vi "sub_LF_params.vi"(6 "error in (no error)":errorcluster, 8 "Numeric":u32, 9 "LightField Automation in":refnum<class "LightField Automation.lvclass">) -> (0 "error out":errorcluster, 2 "Params CCD":string, 3 "LightField Automation out":refnum<class "LightField Automation.lvclass">)   [LabVIEW 2019]
doc: "Runs the Winx32 software trough Labview.\nSoftware trigger with Notifu Winx_Start\nAbort with Notify Winx_Abort\nMade by Wim van Dieren, ImSpec"
uses:
  Ligth Field/lightfield-automation-labview/LightField Automation.lvclass
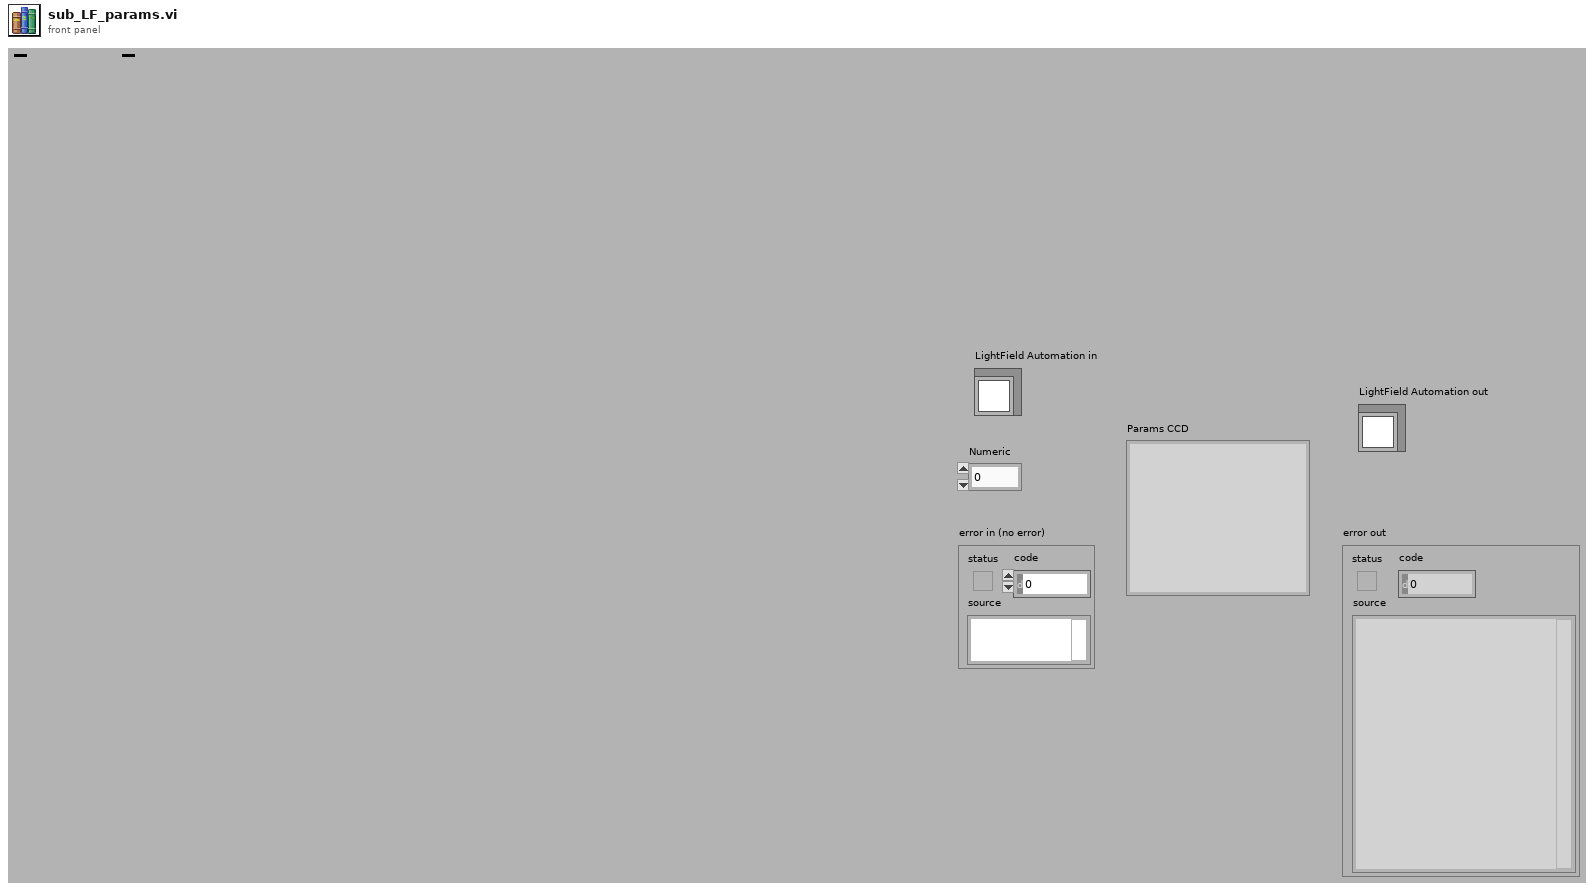
[diagram p1: front panel]
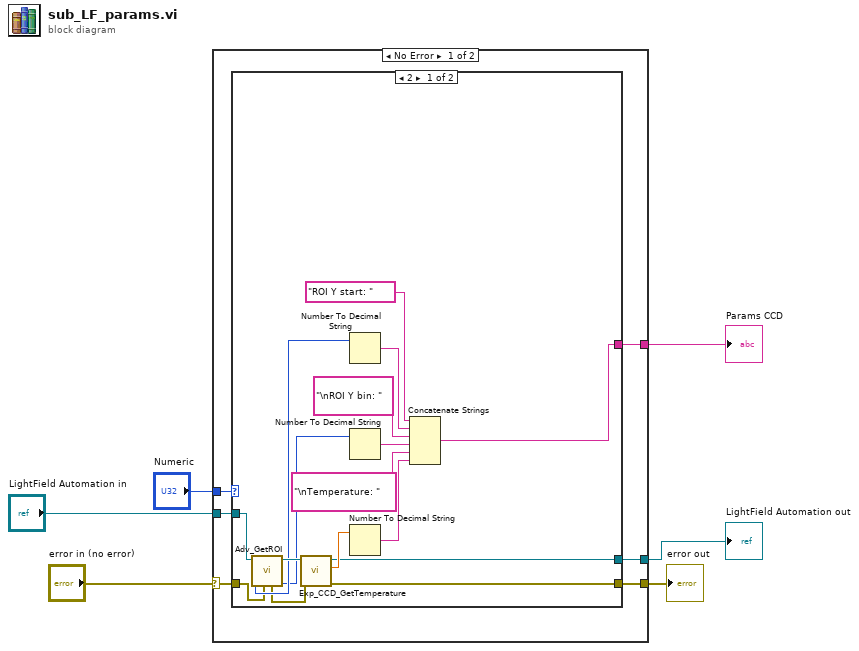
[diagram p0: block diagram]
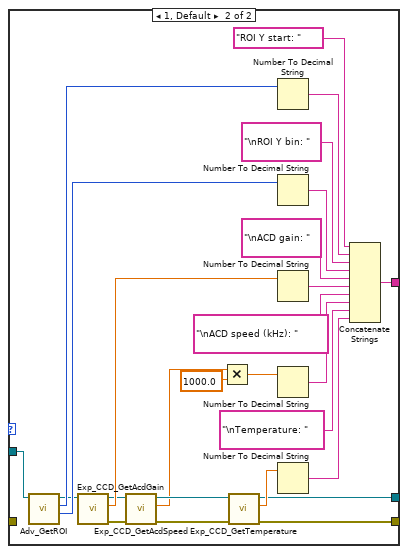
[diagram p2: hidden frame]
diagram:
  n1 = case shown="No Error" "error in (no error)" {
    selector: "error in (no error)" -> [w7 w56]
    tunnel: [w10 w56] -> w5
    tunnel: [w11 w55] -> w3
    tunnel: "LightField Automation in" -> [w12 w55]
    tunnel: [w9 _] -> w2
    tunnel: "Numeric" -> [w8 _]
    frame No Error {
      n2 = case shown="2" w8 {
        tunnel: w12 -> [w23 w36]
        tunnel: [w21 w35] -> w11
        tunnel: [w20 w34] -> w10
        tunnel: [w17 w33] -> w9
        tunnel: w7 -> [w14 _]
        frame 2 {
          n3 = call "Adv_GetROI.vi"("error in (no error)"=w14, "LightField Automation in"=w23) -> ("YBinning"=w15:i32, "LightField Automation out"=w22:refnum<class "LightField Automation.lvclass">, "error out"=w13:errorcluster, "Y"=w16:i32)  [unwired: 2 in, 4 out]
          n4 = call "Exp_CCD_GetTemperature.vi"("error in (no error)"=w13, "LightField Automation in"=w22) -> ("error out"=w20:errorcluster, "Temperature (°C)"=w24:dbl, "LightField Automation out"=w21:refnum<class "LightField Automation.lvclass">)  [unwired: 7 in]
          n5 = Number To Decimal String(number=w16) -> (decimal integer string=w26:string)  [unwired: 1 in]
          n6 = Number To Decimal String(number=w15) -> (decimal integer string=w27:string)  [unwired: 1 in]
          n7 = Number To Decimal String(number=w24) -> (decimal integer string=w18:string)  [unwired: 1 in]
          n8 = Concatenate Strings("ROI Y start: ", w26, "\nROI Y bin: ", w27, "\nTemperature: ", w18) -> (w17:string)
        }
        frame 1, Default {
          n9 = call "Adv_GetROI.vi"("LightField Automation in"=w36) -> ("XBinning"=w53:i32, "Width"=w51:i32, "LightField Automation out"=w50:refnum<class "LightField Automation.lvclass">)  [unwired: 3 in, 5 out]
          n10 = call "Exp_CCD_GetAcdGain.vi"("LightField Automation in"=w50) -> ("error out"=w47:errorcluster, "Gain"=w52:dbl, "LightField Automation out"=w49:refnum<class "LightField Automation.lvclass">)  [unwired: 8 in]
          n11 = call "Exp_CCD_GetAcdSpeed.vi"("error in (no error)"=w47, "LightField Automation in"=w49) -> ("error out"=w46:errorcluster, "Speed (MHz)"=w31:dbl, "LightField Automation out"=w48:refnum<class "LightField Automation.lvclass">)  [unwired: 7 in]
          n12 = Multiply(x=w31, y=1000.0) -> (x*y=w30:dbl)
          n13 = call "Exp_CCD_GetTemperature.vi"("error in (no error)"=w46, "LightField Automation in"=w48) -> ("error out"=w34:errorcluster, "Temperature (°C)"=w54:dbl, "LightField Automation out"=w35:refnum<class "LightField Automation.lvclass">)  [unwired: 7 in]
          n14 = Number To Decimal String(number=w51) -> (decimal integer string=w44:string)  [unwired: 1 in]
          n15 = Number To Decimal String(number=w53) -> (decimal integer string=w42:string)  [unwired: 1 in]
          n16 = Number To Decimal String(number=w52) -> (decimal integer string=w41:string)  [unwired: 1 in]
          n17 = Number To Decimal String(number=w30) -> (decimal integer string=w39:string)  [unwired: 1 in]
          n18 = Number To Decimal String(number=w54) -> (decimal integer string=w37:string)  [unwired: 1 in]
          n19 = Concatenate Strings("ROI Y start: ", w44, "\nROI Y bin: ", w42, "\nACD gain: ", w41, "\nACD speed (kHz): ", w39, "\nTemperature: ", w37) -> (w33:string)
        }
      }
    }
    frame Error {
    }
  }
  "error out" <- w5
  "LightField Automation out" <- w3
  "Params CCD" <- w2
